vi "WILT Check Cycle Index.vi"(8 "error in":errorcluster, 10 "Day":bool, 11 "Cycle Index":string) -> (0 "error out":errorcluster, 2 "Correct Cycle":bool)   [LabVIEW 2016]
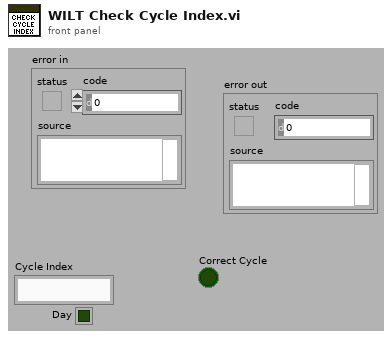
[diagram p1: front panel]
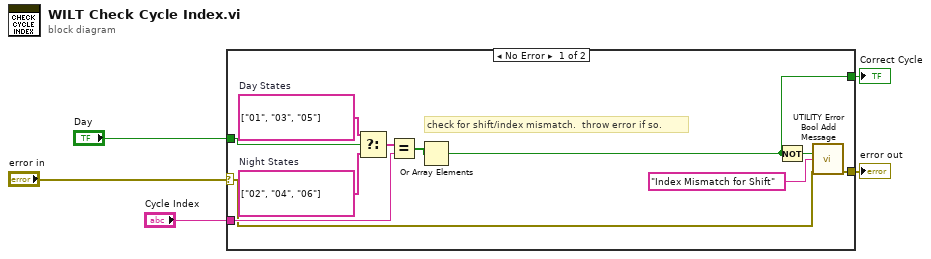
[diagram p0: block diagram]
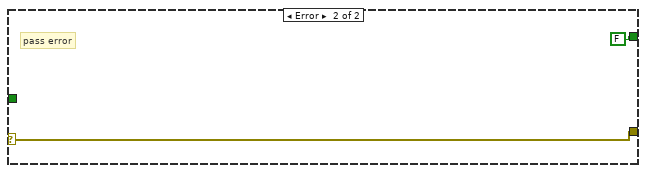
[diagram p2: hidden frame]
diagram:
  n1 = case shown="No Error" "error in" {
    selector: "error in" -> [w10 w18]
    tunnel: [w11 w18] -> w4
    tunnel: "Day" -> [w15 _]
    tunnel: "Cycle Index" -> [w12 _]
    tunnel: [w8 FALSE] -> w1
    frame No Error {
      w7 = string[] ["01", "03", "05"]  # Day States
      w6 = string[] ["02", "04", "06"]  # Night States
      # "check for shift/index mismatch.  throw error if so."
      n2 = Select(t=w7, s=w15, f=w6) -> (s? t:f=w13:string[])
      n3 = Equal?(x=w13, y=w12) -> (x = y?=w14:bool[])
      n4 = Or Array Elements(Boolean array=w14) -> (logical OR=w8:bool)
      n5 = Not(x=w8) -> (.not. x?=w9:bool)
      n6 = call "UTILITY Error Bool Add Message.vi"("Error?"=w9, "Message"="Index Mismatch for Shift", "Error In"=w10) -> ("Error Out"=w11:errorcluster)  [unwired: 12 in]
    }
    frame Error {
      # "pass error"
    }
  }
  "error out" <- w4
  "Correct Cycle" <- w1
